vi "Vision Research Phantom Series PhInt PhMakeColorPAR.vi"(0 "Camera Number (1)":u32=1, 2 "CFA":T1 {"CFA" items=["CFA_NONE", "CFA_VRI", "CFA_VRIV6", "CFA_BAYER", "CFA_BAYERFLIP"]}, 3 "Algorithm":T2=1 items=["FAST_ALGORITHM"=1, "BEST_ALGORITHM"=5, "NO_DEMOSAICING"=6], 4 "pPixel In":u8[](array[numeric]), 5 "Error In (no error)":errorcluster, 7 "BITMAPINFOHEADER":T7) -> (14 "Camera Number out":u32=1, 16 "pPixel":u8[](array[numeric]), 19 "Error Out":errorcluster)   [LabVIEW 2013, in "VRI.lvlib"]
doc: "PhInt.dll\n\nPhMakeColorPAR\nPhMakeColorPAR(int Width, int Height,int BitCount, unsigned char * pPixel, int CFA, int Saturation, int bFlipH, int bFlipV, int Algorithm);\n\nParameters Description\nWidth Image width\nHeight Image height\nBitCount Bits per pixel\npPixel Pixel array pointer\nCFA Color filter array code\nSaturation Color saturation adjustment, –100 …. +100, 0 neutral\nbFlipV Flip Vertical if TRUE\nbFlipH Flip Horizontal if TRUE\nAlgorithm Interpolation algorithm code\nReturn Void\nComments A replacement for LabView of the PhMakeColor function\n\nWritten by:\nBLOOMY CONTROLS, INC\nWINDSOR, CT 06095, USA\n860-298-9925\nwww.bloomy.com\nV1.0.0\nMay, 2004"
uses:
  VRI.lvlib
  _Type Defs/BITMAPINFOHEADER.ctl
  _Type Defs/PhInt WBGAIN.ctl
  _Type Defs/FilterCode.ctl
  _Type Defs/IMFILTER.ctl
  _Type Defs/PhInt Algorithm.ctl
  _Type Defs/PhInt CFA.ctl
  Phantom DLLs/PhInt.Dll
panel:
  in  "IMPROCOPTIONS":T6 {"FilterCode" items=["PREWITT_3X3_V"=1, "PREWITT_3X3_H"=2, "SOBEL_3X3_V"=3, "SOBEL_3X3_H"=4, "LAPLACIAN_3X3"=5, "LAPLACIAN_5X5"=6, "GAUSSIAN_3X3"=7, "GAUSSIAN_5X5"=8, "HIPASS_3x3"=9, "HIPASS_5x5"=10, "SHARPEN_3X3"=11, "USERFILTER"=-1]; "Rotate" min=-90 max=90 step=1; "Saturation" min=-100 max=100 step=1; "Contrast" min=-100 max=100 step=1; "Bright" min=-100 max=100 step=1}
  # "For instructions on the use of this VI, press Ctrl+H to display the help window and move the mouse over the icon, controls, and indicators"
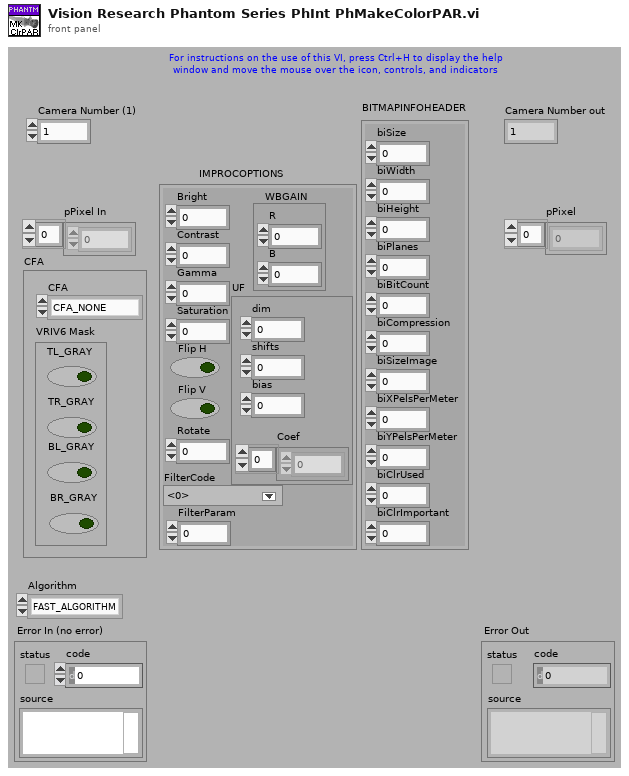
[diagram p1: front panel]
types:
  T1 = typedef "VRI.lvlib/PhInt CFA.ctl" = cluster{"CFA":u32, "VRIV6 Mask":cluster{"TL_GRAY":bool, "TR_GRAY":bool, "BL_GRAY":bool, "BR_GRAY":bool}}
  T2 = typedef "VRI.lvlib/PhInt Algorithm.ctl" = u32
  T3 = typedef "VRI.lvlib/PhInt WBGAIN.ctl" = cluster{"R":sgl, "B":sgl}
  T4 = typedef "VRI.lvlib/FilterCode.ctl" = i32
  T5 = typedef "VRI.lvlib/IMFILTER.ctl" = cluster{"dim":i32, "shifts":i32, "bias":i32, "Coef":i32[]}
  T6 = cluster{"Bright":i32, "Contrast":i32, "Gamma":sgl, "Saturation":i32, "Flip H":bool, "Flip V":bool, "Rotate":i32, "WBGAIN":T3, "FilterCode":T4, "FilterParam":i32, "UF":T5}
  T7 = typedef "VRI.lvlib/BITMAPINFOHEADER.ctl" = cluster{"biSize":u32, "biWidth":i32, "biHeight":i32, "biPlanes":u16, "biBitCount":u16, "biCompression":u32, "biSizeImage":u32, "biXPelsPerMeter":i32, "biYPelsPerMeter":i32, "biClrUsed":u32, "biClrImportant":u32}
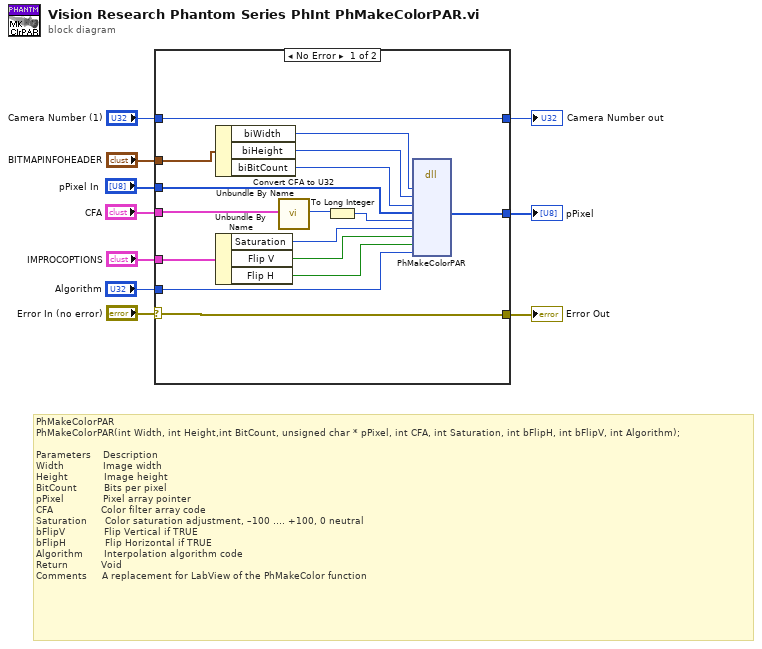
[diagram p0: block diagram]
diagram:
  # "PhMakeColorPAR\nPhMakeColorPAR(int Width, int Height,int BitCount, unsigned char * pPixel, int CFA, int Saturation, int bFlipH, int bFlipV, int Algorithm);\n\nParameters    Description\nWidth             Image width\nHeight            Image height\nBitCount         Bits per pixel\npPixel             Pixel array pointer\nCFA                Color filter array code\nSaturation      Color saturation adjustment, –100 …. +100, 0 neutral\nbFlipV             Flip Vertical if TRUE\nbFlipH             Flip Horizontal if TRUE\nAlgorithm       Interpolation algorithm code\nReturn           Void\nComments     A replacement for LabView of the PhMakeColor function"
  n1 = case shown="No Error" "Error In (no error)" {
    selector: "Error In (no error)" -> [w26 w29]
    tunnel: [w26 w29] -> w9
    tunnel: "Camera Number (1)" -> [w25 w28]
    tunnel: [w25 w28] -> w7
    tunnel: "BITMAPINFOHEADER" -> [w24 _]
    tunnel: [w23 w27] -> w5
    tunnel: "IMPROCOPTIONS" -> [w22 _]
    tunnel: "CFA" -> [w21 _]
    tunnel: "Algorithm" -> [w20 _]
    tunnel: "pPixel In" -> [w19 w27]
    frame No Error {
      n2 = Unbundle By Name(w24) -> ("biWidth"=w18:i32, "biHeight"=w17:i32, "biBitCount"=w16:u16)
      n3 = Unbundle By Name(w22) -> ("Saturation"=w13:i32, "Flip V"=w14:bool, "Flip H"=w15:bool)
      n4 = call "Convert CFA to U32.vi"("CFA in"=w21) -> ("CFA out"=w12:u32)  [unwired: 18 out]
      n5 = To Long Integer(number=w12) -> (32bit integer=w11:i32)
      n6 = dll-call lib="C:/Projects/SDK/64-bit/Vision Research Phantom Series Labview Driver/Phantom DLLs/PhInt.dll" fn="PhMakeColorPAR"("Width"=w18, "Height"=w17, "BitCount"=w16, "pPixel"=w19, "CFA"=w11, "Saturation"=w13, "FlipV"=w14, "FlipH"=w15, "Algorithm"=w20) -> ("pPixel"=w23:u8[])  [unwired: 9 in, 5 out]
    }
    frame Error {
    }
  }
  "Error Out" <- w9
  "Camera Number out" <- w7
  "pPixel" <- w5
